vi "all-quintic-spline-test.vi"() -> (3 "ALL TESTS PASSED":bool)   [LabVIEW 2019]
panel:
  out "Test 6":bool
  out "Test 5":bool
  out "Test 4":bool
  out "Test 3B":bool
  out "Test 3A":bool
  out "Test 2":bool
  out "Test 1":bool
  out "Test 0":bool
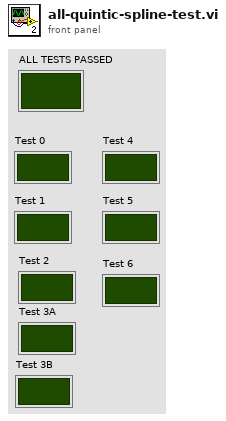
[diagram p1: front panel]
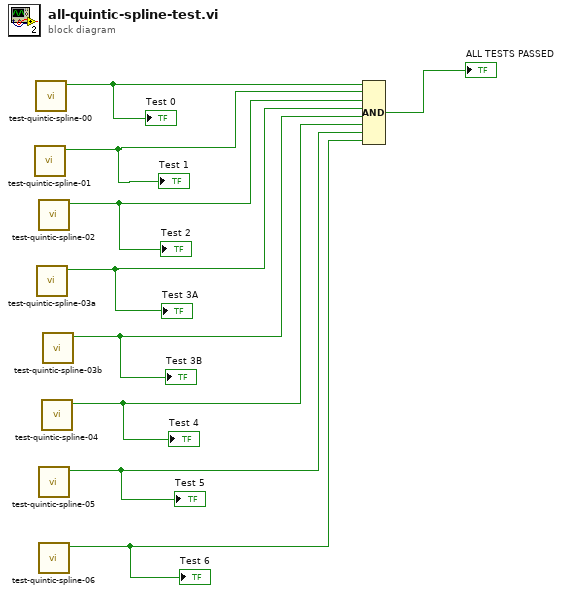
[diagram p0: block diagram]
diagram:
  n1 = call "test-quintic-spline-01.vi"() -> ("Test Passed"=w7:bool)  [unwired: 11 in]
  "Test 1" <- w7
  n2 = call "test-quintic-spline-00.vi"() -> ("Test Passed"=w8:bool)  [unwired: 11 in]
  "Test 0" <- w8
  n3 = call "test-quintic-spline-03a.vi"() -> ("Test Passed"=w4:bool)  [unwired: 11 in]
  "Test 3A" <- w4
  n4 = call "test-quintic-spline-02.vi"() -> ("Test Passed"=w6:bool)  [unwired: 11 in]
  "Test 2" <- w6
  n5 = call "test-quintic-spline-05.vi"() -> ("Test Passed"=w2:bool)  [unwired: 11 in]
  "Test 5" <- w2
  n6 = call "test-quintic-spline-06.vi"() -> ("Test Passed"=w1:bool)  [unwired: 11 in]
  "Test 6" <- w1
  n7 = call "test-quintic-spline-04.vi"() -> ("Test Passed"=w3:bool)  [unwired: 11 in]
  "Test 4" <- w3
  n8 = call "test-quintic-spline-03b.vi"() -> ("Test Passed"=w5:bool)  [unwired: 11 in]
  "Test 3B" <- w5
  n9 = Compound Arithmetic op=AND(w8, w7, w6, w4, w5, w3, w2, w1) -> (→"ALL TESTS PASSED":bool)
